vi "Run.vi"(7 "Team Index":i32, 8 "Column":i32, 9 "Row":i32, 10 "View":i32[](array[numeric]) caption="View (Team Index, -1: empty)", 11 "Experience In":refnum<class "Experience.lvclass">) -> (0 "Replicated":refnum<class "Square.lvclass">, 1 "Direction":T1, 2 "Action":T2, 3 "Square Out":refnum<class "Square.lvclass">)   [LabVIEW 2015, in "Experience.lvclass"]
uses:
  Experience.lvclass
  Square/Square.lvclass
  Type Defs/Action Enum.ctl
  Type Defs/Direction Enum.ctl
  Experience.lvclass/Experience.ctl
  Data Cluster.ctl
  SubVIs/Read-Only Globals.vi
  SubVIs/Globals (private).vi
  <vilib>/ActorFramework/Reply Msg/Reply Msg.lvclass
  <vilib>/ActorFramework/Stop Msg/Stop Msg.lvclass
  <vilib>/ActorFramework/Actor/Actor.lvclass
  Type Defs/SB Type Defs.lvlib
panel:
  # "NW\nN\nNE\nE\nSE\nS\nSW\nW"
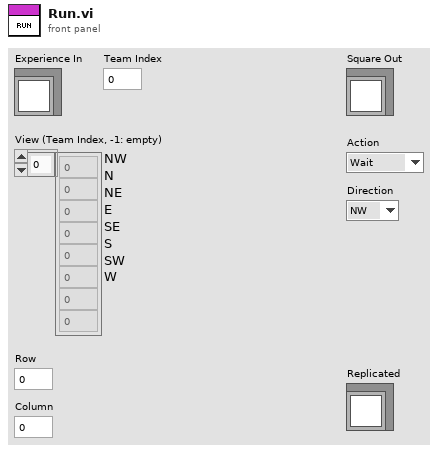
[diagram p1: front panel]
types:
  T1 = typedef "SB Type Defs.lvlib/Direction Enum.ctl" = enum16{"NW", "N", "NE", "E", "SE", "S", "SW", "W"}
  T2 = typedef "SB Type Defs.lvlib/Action Enum.ctl" = enum16{"Wait", "Move", "Attack", "Replicate"}
  T3 = typedef "Experience.lvclass/Data Cluster.ctl" = cluster{"Field":u8[][]}
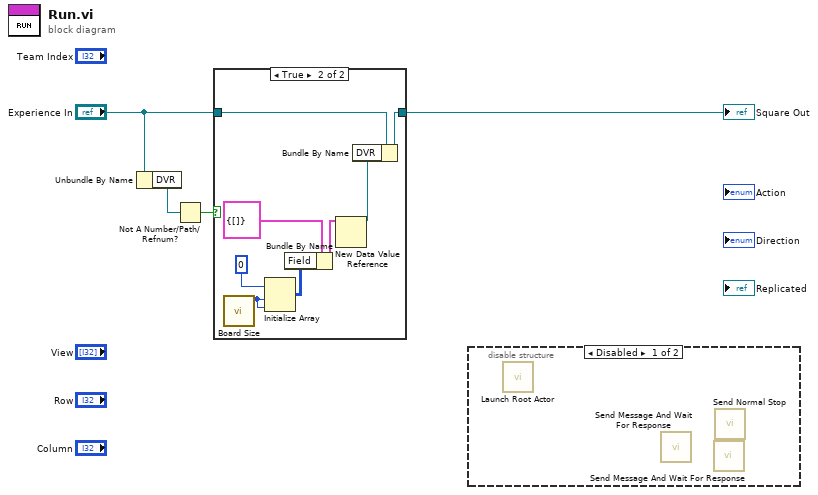
[diagram p0: block diagram]
diagram:
  n1 = Unbundle By Name("Experience In") -> ("DVR"=w4:refnum<data-value>)
  n2 = Not A Number/Path/Refnum?(number/path/refnum=w4) -> (NaN/Path/Refnum?=w3:bool)
  n3 = case shown="True" w3 {
    tunnel: "Experience In" -> [w5 w11]
    tunnel: [w5 w10] -> w1
    frame False {
    }
    frame True {
      n4 = call "Board Size.vi"() -> ("Board Size"=w8:i32)  [unwired: 11 in]
      n5 = Initialize Array(u8 0, w8, w8) -> (w7:u8[][])
      n6 = Bundle By Name(cluster=T3 {"Field"=[]} ("Data"), "Field"=w7) -> (w12:T3)
      n7 = New Data Value Reference(data value=w12) -> (data value reference=w6:refnum<data-value>)  [unwired: 1 in, 1 out]
      n8 = Bundle By Name(cluster=w11, "DVR"=w6) -> (w10:refnum<class "Experience.lvclass">)
    }
  }
  "Square Out" <- w1
  n9 = disable-structure shown="Disabled" {
    frame Disabled {
      n10 = call <vilib>:"Launch Root Actor.vi"() -> ()  [unwired: 10 in, 2 out]
      n11 = call <vilib>:"Send Message And Wait For Response.vi"() -> ()  [unwired: 8 in, 4 out]
      n12 = call <vilib>:"Send Message And Wait For Response.vi"() -> ()  [unwired: 8 in, 4 out]
      n13 = call <vilib>:"Send Normal Stop.vi"() -> ()  [unwired: 11 in, 1 out]
    }
    frame Enabled {
    }
  }
